vi "Host_FastOsziTest_3Ghz.vi"() -> ()   [LabVIEW 2014]
uses:
  <vilib>/FPGAPlugInAG/PXIe-7962R/niLvFpga_Open_PXIe-7962R.vi
  <vilib>/rvi/interface/common/dynamic/niFpgaDynamicAddResources.vi
  <vilib>/Utility/error.llb/Error Cluster From Error Code.vi
  <vilib>/rvi/errors/niLvFpgaAdjustHostInterfaceError.vi
  <vilib>/FPGAPlugInAG/Dynamic/niLvFpga_Close_Dynamic.vi
  <vilib>/rvi/interface/nirviOpenFPGA/nirviOpenFPGA.xnode
  Scope/fpga_labview/FPGA Bitfiles/AnalogIntegratorFastOszi_NI5771_PXIe-7962R.lvbitx
  <vilib>/rvi/interface/nirviReadWriteControl/nirviReadWriteControl.xnode
  <vilib>/rvi/interface/nirviMethod/nirviMethod.xnode
  <vilib>/rvi/interface/nirviCloseFPGA/nirviCloseFPGA.xnode
  <vilib>/rvi/interface/Simulation/niFpgaSimulationCallBeginRW.vi
  NiFpgaLv.dll
  <vilib>/FPGAPlugInAG/Dynamic/niLvFpga_ReadFifo_Dynamic.vi
  <vilib>/rvi/errors/niLvFpgaMergeErrorWithErrorCode.vi
  <vilib>/Analysis/NI_AALPro.lvlib
panel:
  out "User Command Status":u8=16
  in  "Repetition Rate":bool=TRUE
  in  "Baseline Subtract":u8=16
  out "NOT Crosstalk":dbl format="%0.2f"
  out "Crosstalk":dbl format="%0.2f"
  in  "Save?":bool
  out "time to draw(ms) 2":i32=1000
  out "Area 1":picture
  in  "sized scatter plot cosmetics 2":T1={"min size"=1, "max size"=5, "maps to max size"=5, "color array"=[16711680, 65280, 255, 16776960, 16737792, 65535]}
  in  "cartesian axis attributes 2":T2={"x minimum"=1.0, "x maximum"=500.0, "x log?"=FALSE, "x precision"=1, "x format"=enum."Decimal", "y minimum"=60.0, "y maximum"=740.0, "y log?"=FALSE, "y precision"=1, "y format"=enum."Decimal"} {"x minimum" format="%0.2f"; "x maximum" format="%0.2f"; "y minimum" format="%0.2f"; "y maximum" format="%0.2f"}
  in  "?":u16(ring)=4 items=["Points", "Squares", "Circles", "Sized Squares", "Sized-Colored Squares", "Min-Max Lines"]
  in  "line color 2":u32(colorbox)=39168
  in  "text color 2":u32(colorbox)=65280
  in  "plot color 2":u32(colorbox)=16776960
  out "time to draw(ms)":i32=1000
  out "Area 2":picture
  in  "sized scatter plot cosmetics":T1={"min size"=1, "max size"=5, "maps to max size"=5, "color array"=[16711680, 65280, 255, 16776960, 16737792, 65535]}
  in  "cartesian axis attributes":T2={"x minimum"=1.0, "x maximum"=500.0, "x log?"=FALSE, "x precision"=1, "x format"=enum."Decimal", "y minimum"=60.0, "y maximum"=740.0, "y log?"=FALSE, "y precision"=1, "y format"=enum."Decimal"} {"x minimum" format="%0.2f"; "x maximum" format="%0.2f"; "y minimum" format="%0.2f"; "y maximum" format="%0.2f"}
  in  "?":u16(ring)=4 items=["Points", "Squares", "Circles", "Sized Squares", "Sized-Colored Squares", "Min-Max Lines"]
  in  "line color":u32(colorbox)=39168
  in  "text color":u32(colorbox)=65280
  in  "plot color":u32(colorbox)=16776960
  out "PMT histogram":T3(graph)
  out "Mean NOT pulse length":dbl format="%0.2f"
  out "Mean pulse length":dbl format="%0.2f"
  out "NOT Laser pulse length histogram":T3(graph)
  out "Laser pulse length histogram":T3(graph)
  out "Laser (Trigger In)":i16[](graph)
  in  "Samples per Pixels":u32=10000
  out "IO Module\\AI Over Range":bool
  out "PMT (AI 0)":u8[](graph)
  # "Sampling at 1.5GHz => 0.66 ns sampling interval"
  # "40MHz"
  # "80MHz"
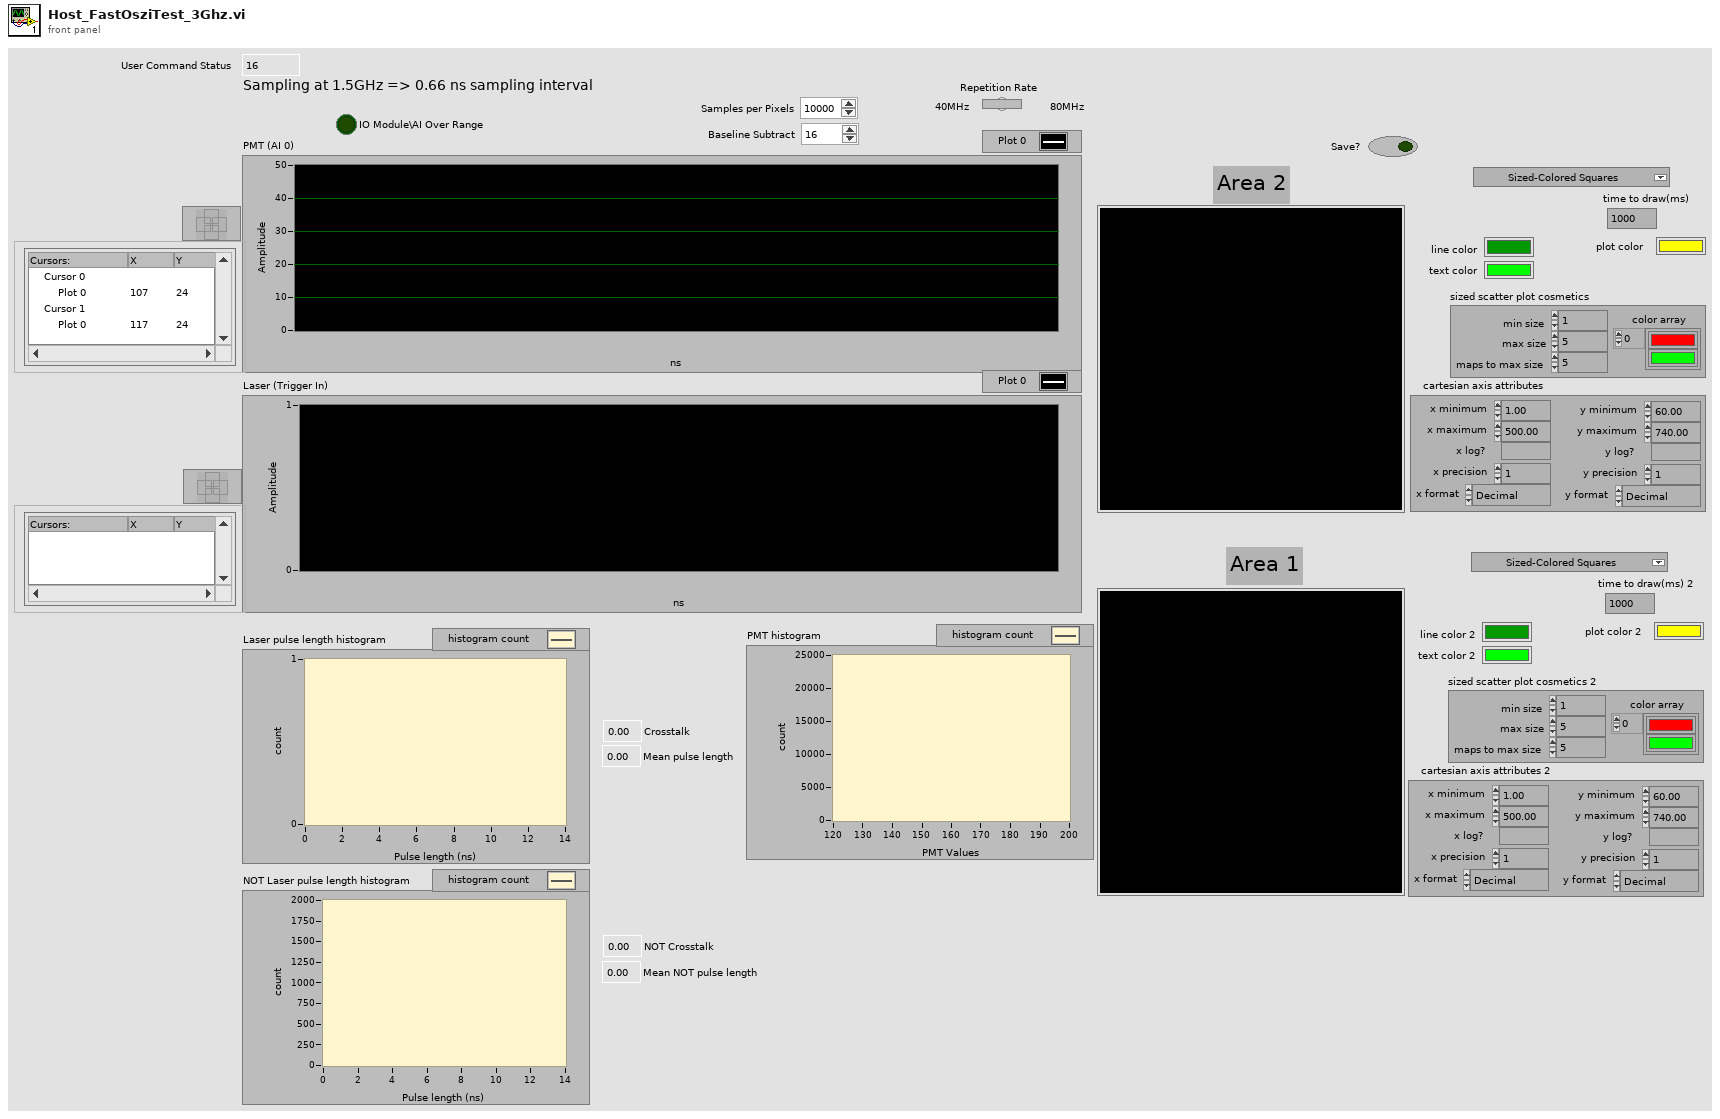
[diagram p1: front panel]
types:
  T1 = cluster{"min size":i16, "max size":i16, "maps to max size":i16, "color array":u32[]}
  T2 = cluster{"x minimum":dbl, "x maximum":dbl, "x log?":bool, "x precision":u8, "x format":enum8{"Decimal", "Scientific", "Engineering", "Binary", "Octal", "Hex"}, "y minimum":dbl, "y maximum":dbl, "y log?":bool, "y precision":u8, "y format":enum8{"Decimal", "Scientific", "Engineering", "Binary", "Octal", "Hex"}}
  T3 = cluster{"X Values":dbl[], "Histogram: h(x)":i32[]}
  T4 = typedef "LVBoundsTypeDef.ctl" = cluster{"Width":u32, "Height":u32}
  T5 = cluster{"line color 2":u32, "text color 2":u32, "tick length":i16, "not crossing axes":bool, "no grids":bool}
  T6 = cluster{"plot color 2":u32, i32, "baseline(not used for these plots)":i16}
  T7 = cluster{cluster{i32, i32, "Width":u32, "Height":u32}, "cartesian axis attributes 2":cluster{"x minimum":dbl, "x maximum":dbl, "x log?":bool, "x precision":u8, "x format":enum8{"Decimal", "Scientific", "Engineering", "Binary", "Octal", "Hex"}, "y minimum":dbl, "y maximum":dbl, "y log?":bool, "y precision":u8, "y format":enum8{"Decimal", "Scientific", "Engineering", "Binary", "Octal", "Hex"}}, cluster{"line color 2":u32, "text color 2":u32, "tick length":i16, "not crossing axes":bool, "no grids":bool}, cluster{"plot color 2":u32, i32, "baseline(not used for these plots)":i16}, "sized scatter plot cosmetics 2":cluster{"min size":i16, "max size":i16, "maps to max size":i16, "color array":u32[]}}
  T8 = cluster{"line color":u32, "text color":u32, "tick length":i16, "not crossing axes":bool, "no grids":bool}
  T9 = cluster{"plot color":u32, i32, "baseline(not used for these plots)":i16}
  T10 = cluster{cluster{i32, i32, "Width":u32, "Height":u32}, "cartesian axis attributes":cluster{"x minimum":dbl, "x maximum":dbl, "x log?":bool, "x precision":u8, "x format":enum8{"Decimal", "Scientific", "Engineering", "Binary", "Octal", "Hex"}, "y minimum":dbl, "y maximum":dbl, "y log?":bool, "y precision":u8, "y format":enum8{"Decimal", "Scientific", "Engineering", "Binary", "Octal", "Hex"}}, cluster{"line color":u32, "text color":u32, "tick length":i16, "not crossing axes":bool, "no grids":bool}, cluster{"plot color":u32, i32, "baseline(not used for these plots)":i16}, "sized scatter plot cosmetics":cluster{"min size":i16, "max size":i16, "maps to max size":i16, "color array":u32[]}}
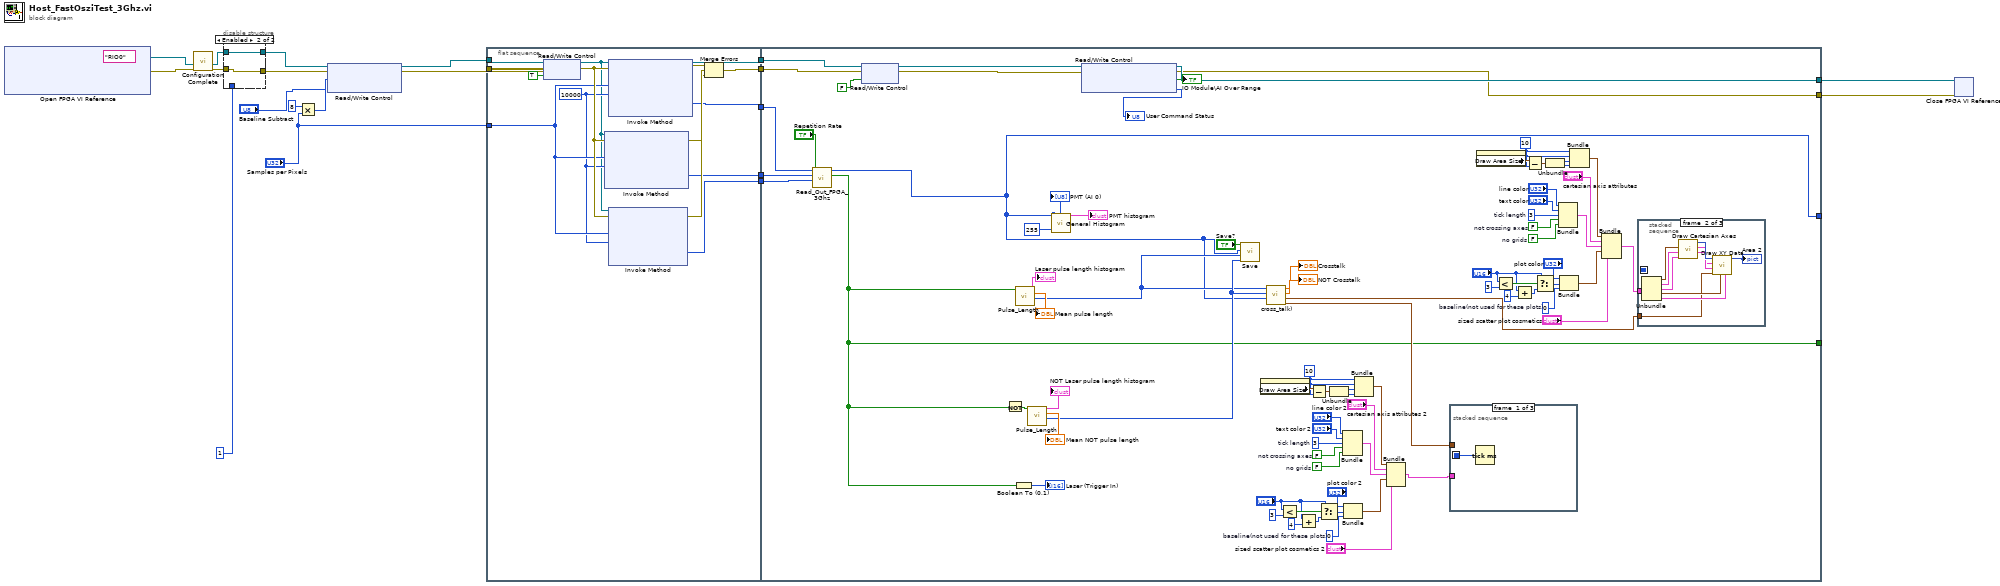
[diagram p0: block diagram]
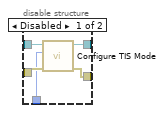
[diagram p2: hidden frame]
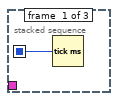
[diagram p3: hidden frame]
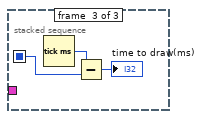
[diagram p4: hidden frame]
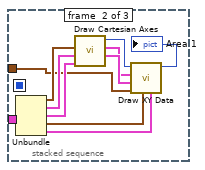
[diagram p5: hidden frame]
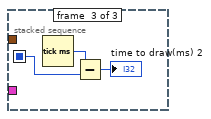
[diagram p6: hidden frame]
diagram:
  n1 = xnode "Open FPGA VI Reference"("resource name"=tag "RIO0") -> ("FPGA VI Reference Out"=w7:refnum<k20>, "error out"=w20:errorcluster)  [unwired: 1 in]
  n2 = call "Configuration Complete.vi"("error in"=w20, "FPGA VI Reference In 2"=w7) -> ("error out"=w4:errorcluster, "FPGA VI Reference Out 2"=w5:refnum<k20>)  [unwired: 6 in, 2 out]
  n3 = disable-structure shown="Enabled" {
    disable-tunnel: w5 -> [w26 w27]
    disable-tunnel: w4 -> [w25 w28]
    disable-tunnel: [w24 w28] -> w3
    disable-tunnel: [w23 w27] -> w2
    disable-tunnel: 1 -> [w22 _]
    frame Disabled {
      n4 = call "Configure TIS Mode.vi"("error in"=w25, "AI Channel"=w22, "FPGA VI Reference In 2"=w26) -> ("error out"=w24:errorcluster, "FPGA VI Reference Out 2"=w23:refnum<k20>)  [unwired: 6 in, 1 out]
    }
    frame Enabled {
    }
  }
  n5 = Multiply(x=u32 8, y="Samples per Pixels") -> (x*y=w14:u32)
  n6 = xnode "Read/Write Control"("FPGA VI Reference In"=w2, "error in"=w3, "Samples to acquire"=w14, "Baseline U8"="Baseline Subtract") -> ("FPGA VI Reference Out"=w18:refnum<k20>, "error out"=w19:errorcluster)
  n7 = flat-sequence {
    tunnel: w19 -> [w38]
    tunnel: w18 -> [w40]
    tunnel: [w39] -> w11
    tunnel: [w36] -> w10
    tunnel: [w37] -> w9
    tunnel: [w35] -> w8
    tunnel: "Samples per Pixels" -> [w32]
    tunnel: [w31] -> w6
    tunnel: [w121] -> w17
    tunnel: [w120] -> w16
    tunnel: [w45] -> _
    tunnel: [w46] -> _
    tunnel: w11 -> [w117]
    tunnel: w10 -> [w50]
    tunnel: w9 -> [w118]
    tunnel: w8 -> [w48]
    tunnel: w6 -> [w49]
    frame #0 {
      w30 = 10000 ("Timeout (ms)")
      n8 = xnode "Read/Write Control"("FPGA VI Reference In"=w40, "error in"=w38, "Acquire"=TRUE) -> ("FPGA VI Reference Out"=w29:refnum<k20>, "error out"=w33:errorcluster)
      n9 = xnode "Invoke Method"("FPGA VI Reference In"=w29, "error in"=w33, "Number of Elements"=w32, "Timeout (ms)"=w30) -> ("error out"=w34:errorcluster, "Data"=w31:u64[])  [unwired: 2 out]
      n10 = xnode "Invoke Method"("FPGA VI Reference In"=w29, "error in"=w33, "Number of Elements"=w32, "Timeout (ms)"=w30) -> ("FPGA VI Reference Out"=w39:refnum<k20>, "error out"=w42:errorcluster, "Data"=w36:u64[])  [unwired: 1 out]
      n11 = xnode "Invoke Method"("FPGA VI Reference In"=w29, "error in"=w33, "Number of Elements"=w32, "Timeout (ms)"=w30) -> ("error out"=w43:errorcluster, "Data"=w35:u8[])  [unwired: 2 out]
      n12 = Merge Errors(w42, w43, w34) -> (w37:errorcluster)
    }
    frame #1 {
      w60 = i16 0  # baseline(not used for these plots)
      w67 = FALSE  # not crossing axes
      w68 = i16 3  # tick length
      w66 = FALSE  # no grids
      w71 = 10
      w83 = i16 0  # baseline(not used for these plots)
      w90 = FALSE  # not crossing axes
      w91 = i16 3  # tick length
      w89 = FALSE  # no grids
      w94 = 10
      n13 = call "Read_Out_FPGA_3Ghz.vi"("Repetition Rate"="Repetition Rate", "U8ReadFIFO"=w48, "U64ReadFIFO 2"=w49, "U64ReadFIFO1"=w50) -> ("Trigger"=w46:bool[], "PMT Signal"=w45:u8[])  [unwired: 6 in]
      "PMT (AI 0)" <- w45
      n14 = xnode "Read/Write Control"("FPGA VI Reference In"=w117, "error in"=w118, "Acquire"=FALSE) -> ("FPGA VI Reference Out"=w115:refnum<k20>, "error out"=w116:errorcluster)
      n15 = Not(x=w46) -> (.not. x?=w112:bool[])
      n16 = Boolean To (0,1)(Boolean=w46) -> (0, 1=→"Laser (Trigger In)":i16[])
      n17 = call "Pulse_Length.vi"("Trigger"=w46) -> ("Rising Index"=w101:i32[], "Mean Pulse Length"=→"Mean pulse length":dbl, "Histogram Graph"=→"Laser pulse length histogram":T3)  [unwired: 8 in]
      n18 = call "Pulse_Length.vi"("Trigger"=w112) -> ("Rising Index"=w104:i32[], "Mean Pulse Length"=→"Mean NOT pulse length":dbl, "Histogram Graph"=→"NOT Laser pulse length histogram":T3)  [unwired: 8 in]
      n19 = call <vilib>:"General Histogram.vi"("X"=w45, "# bins"=255) -> ("Histogram Graph"=→"PMT histogram":T3)  [unwired: 9 in, 4 out]
      n20 = xnode "Read/Write Control"("FPGA VI Reference In"=w115, "error in"=w116) -> ("FPGA VI Reference Out"=w121:refnum<k20>, "error out"=w120:errorcluster, "IO Module\\AI Over Range"=→"IO Module\\AI Over Range":bool, "User Command Status"=→"User Command Status":u8)
      n21 = call "Save.vi"("Rising Index 1"=w104, "Rising Index 2"=w101, "PMT (AI 0)"=w45, "Save?"="Save?") -> ()  [unwired: 8 in]
      n22 = property on="Area 1" class="Pict"() -> ("Draw Area Size"=w98:T4)  [unwired: 2 in, 2 out]
      n23 = call "cross_talk).vi"("Array"=w45, "Rising Index 2"=w104, "Rising Index"=w101) -> ("data 2"=w100:cluster{"x":dbl, "y":dbl}[], "data"=w99:cluster{"x":dbl, "y":dbl}[], "x/y 2"=→"NOT Crosstalk":dbl, "x/y"=→"Crosstalk":dbl)  [unwired: 5 in]
      n24 = Less?(x="?", y=3) -> (x < y?=w88:bool)
      n25 = Add(x="?", y=4) -> (x+y=w86:i32)
      n26 = Subtract(x=w98, y=w94) -> (x-y=w97:T4)
      n27 = Select(t="?", s=w88, f=w86) -> (s? t:f=w84:i32)
      n28 = Unbundle(w97) -> ("Width"=w95:u32, "Height"=w96:u32)
      n29 = Bundle("line color 2"="line color 2", "text color 2"="text color 2", "tick length"=w91, "not crossing axes"=w90, "no grids"=w89) -> (w78:T5)  [unwired: 1 in]
      n30 = Bundle("plot color 2"="plot color 2", w84, "baseline(not used for these plots)"=w83) -> (w79:T6)  [unwired: 1 in]
      n31 = Bundle(w94, w94, "Width"=w95, "Height"=w96) -> (w76:cluster{i32, i32, "Width":u32, "Height":u32})  [unwired: 1 in]
      n32 = Bundle(w76, "cartesian axis attributes 2"="cartesian axis attributes 2", w78, w79, "sized scatter plot cosmetics 2"="sized scatter plot cosmetics 2") -> (w52:T7)  [unwired: 1 in]
      n33 = stacked-sequence {
        seq-local: [w137 _ _] -> [_ _ w150]
        tunnel: w52 -> [_ w142 _]
        tunnel: w100 -> [_ w138 _]
        frame #0 {
          n34 = Tick Count (ms)() -> (millisecond timer value=w137:u32)
        }
        frame #1 {
          n35 = Unbundle(w142) -> (w143:cluster{i32, i32, "Width":u32, "Height":u32}, "cartesian axis attributes 2"=w144:T2, w145:T5, w140:T6, "sized scatter plot cosmetics 2"=w139:T1)
          n36 = call <vilib>:"Draw Cartesian Axes.vi"("grid cosmetics"=w145, "axis attributes"=w144, "bounding rect"=w143) -> ("y scale factors"=w147:cluster{"a":dbl, "b":dbl, "log?":bool}, "x scale factors"=w146:cluster{"a":dbl, "b":dbl, "log?":bool}, "new picture"=w148:picture)  [unwired: 6 in]
          n37 = call <vilib>:"Draw XY Data.vi"("[sized scatter plot cosmetics]"=w139, "xy cosmetics"=w140, "xy data"=w138, "y scale factors"=w147, "x scale factors"=w146, "picture"=w148) -> ("new picture"=→"Area 1":picture)  [unwired: 5 in]
        }
        frame #2 {
          n38 = Tick Count (ms)() -> (millisecond timer value=w151:u32)
          n39 = Subtract(x=w151, y=w150) -> (x-y=→"time to draw(ms) 2":u32)
        }
      }
      n40 = property on="Area 2" class="Pict"() -> ("Draw Area Size"=w75:T4)  [unwired: 2 in, 2 out]
      n41 = Less?(x="?", y=3) -> (x < y?=w65:bool)
      n42 = Add(x="?", y=4) -> (x+y=w63:i32)
      n43 = Subtract(x=w75, y=w71) -> (x-y=w74:T4)
      n44 = Select(t="?", s=w65, f=w63) -> (s? t:f=w61:i32)
      n45 = Unbundle(w74) -> ("Width"=w72:u32, "Height"=w73:u32)
      n46 = Bundle("line color"="line color", "text color"="text color", "tick length"=w68, "not crossing axes"=w67, "no grids"=w66) -> (w55:T8)  [unwired: 1 in]
      n47 = Bundle("plot color"="plot color", w61, "baseline(not used for these plots)"=w60) -> (w56:T9)  [unwired: 1 in]
      n48 = Bundle(w71, w71, "Width"=w72, "Height"=w73) -> (w53:cluster{i32, i32, "Width":u32, "Height":u32})  [unwired: 1 in]
      n49 = Bundle(w53, "cartesian axis attributes"="cartesian axis attributes", w55, w56, "sized scatter plot cosmetics"="sized scatter plot cosmetics") -> (w51:T10)  [unwired: 1 in]
      n50 = stacked-sequence {
        seq-local: [w122 _ _] -> [_ _ w135]
        tunnel: w51 -> [_ w127 _]
        tunnel: w99 -> [_ w123 _]
        frame #0 {
          n51 = Tick Count (ms)() -> (millisecond timer value=w122:u32)
        }
        frame #1 {
          n52 = Unbundle(w127) -> (w128:cluster{i32, i32, "Width":u32, "Height":u32}, "cartesian axis attributes"=w129:T2, w130:T8, w125:T9, "sized scatter plot cosmetics"=w124:T1)
          n53 = call <vilib>:"Draw Cartesian Axes.vi"("grid cosmetics"=w130, "axis attributes"=w129, "bounding rect"=w128) -> ("y scale factors"=w132:cluster{"a":dbl, "b":dbl, "log?":bool}, "x scale factors"=w131:cluster{"a":dbl, "b":dbl, "log?":bool}, "new picture"=w133:picture)  [unwired: 6 in]
          n54 = call <vilib>:"Draw XY Data.vi"("[sized scatter plot cosmetics]"=w124, "xy cosmetics"=w125, "xy data"=w123, "y scale factors"=w132, "x scale factors"=w131, "picture"=w133) -> ("new picture"=→"Area 2":picture)  [unwired: 5 in]
        }
        frame #2 {
          n55 = Tick Count (ms)() -> (millisecond timer value=w136:u32)
          n56 = Subtract(x=w136, y=w135) -> (x-y=→"time to draw(ms)":u32)
        }
      }
    }
  }
  n57 = xnode "Close FPGA VI Reference"("FPGA VI Reference In"=w17, "error in"=w16) -> ()  [unwired: 1 out]
